vi "thermistor transfer function OLD.vi"(8 "R_inf":fxp<+/-,32,16>, 9 "B":fxp<+/-,32,16>, 10 "R":fxp<+/-,32,16>) -> ()   [LabVIEW 2018]
uses:
  <vilib>/rvi/FXPMathLib/FxpDiv/subVIs/nifxpmath_Div_SimConfig.ctl
  <vilib>/rvi/FXPMathLib/FxpDiv/simVIs/DllFxpDivTemp_sub.vi
  <vilib>/rvi/FXPMathLib/FxpDiv/XNode/nifxpmath_Div.xnode
  <vilib>/rvi/FXPMathLib/FxpSub/XNode/nifxpmath_Sub.xnode
  <vilib>/rvi/FXPMathLib/sim/FxpSim.dll
panel:
  in  "ready for output (T)":bool=TRUE
  out "Temperature":fxp<+/-,32,16>
  out "output valid":bool
  in  "input valid":bool=TRUE
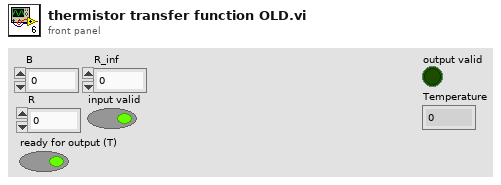
[diagram p1: front panel]
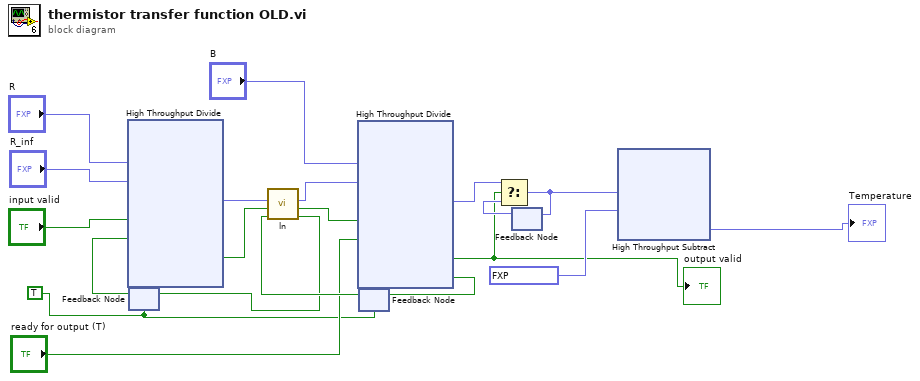
[diagram p0: block diagram]
diagram:
  w5 = TRUE
  n1 = feedback #1(w5) -> (w17:bool)
  n2 = xnode "High Throughput Divide"("x"="R", "y"="R_inf", "input valid"="input valid", "ready for output (T)"=w17) -> ("x/y"=w20:fxp<+/-,64,32>, "output valid"=w18:bool)  [unwired: 1 out]
  n3 = feedback #2(w5) -> (w15:bool)
  n4 = call "ln.vi"("ready for output (T)"=w15, "input valid"=w18, "x"=w20) -> ("ready for input"=w14:bool, "output valid"=w9:bool, "ln(x)"=w19:fxp<+/-,32,16>)  [unwired: 6 in]
  n5 = feedback-in #1(w14) -> ()
  n6 = xnode "High Throughput Divide"("x"="B", "y"=w19, "input valid"=w9, "ready for output (T)"="ready for output (T)") -> ("x/y"=w7:fxp<+/-,32,16>, "output valid"=w1:bool, "ready for input"=w16:bool)
  "output valid" <- w1
  n7 = feedback-in #2(w16) -> ()
  n8 = feedback #3() -> (w6:fxp<+/-,32,16>)  [unwired: 1 in]
  n9 = Select(t=w7, s=w1, f=w6) -> (s? t:f=w4:fxp<+/-,32,16>)
  n10 = feedback-in #3(w4) -> ()
  n11 = xnode "High Throughput Subtract"("x"=w4, "y"=fxp<+,16,9> 273.1484375) -> ("x-y"=→"Temperature":fxp<+/-,32,16>)
